vi "Configure Jitter Measurement (Clock TIE).vi"(6 "Clock TIE Slope (0: Rising)":u16(ring) items=["Rising", "Falling", "Both"], 8 "error in (no error)":errorcluster, 9 "Clock TIE Units (0: Seconds)":u16(ring) items=["Seconds", "Unit Interval"], 10 "Clock TIE Source (0: Channel 1)":u16(ring) items=["Channel 1", "Channel 2", "Channel 3", "Channel 4", "Math 1", "Math 2", "Math 3", "Math 4", "Reference Waveform 1", "Reference Waveform 2", "Reference Waveform 3", "Reference Waveform 4"], 11 "VISA resource name":refnum<visa-resource-name>) -> (0 "error out":errorcluster, 3 "VISA resource name out":refnum<visa-resource-name>)   [LabVIEW 2023, in "Keysight-DSQx3014T.lvlib"]
doc: "Enables Jitter Analysis and configures the Clock TIE (Time Interval Error) jitter measurement which compares edges in a clock signal with the edges in an ideal clock signal determined by the clock recovery feature.\n\n<b>Note:</b>\nThis VI is specific to the 6000-X Series oscilloscopes. These features are not available on other models."
uses:
  Keysight-DSQx3014T.lvlib
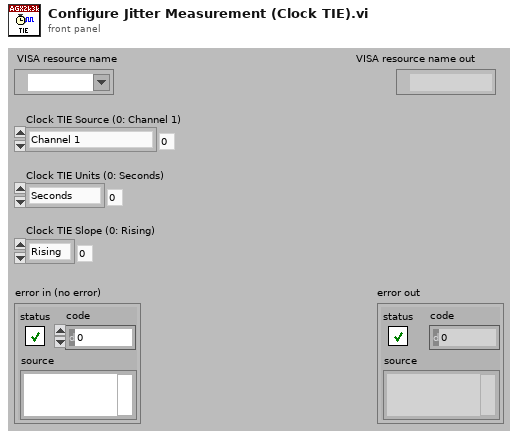
[diagram p1: front panel]
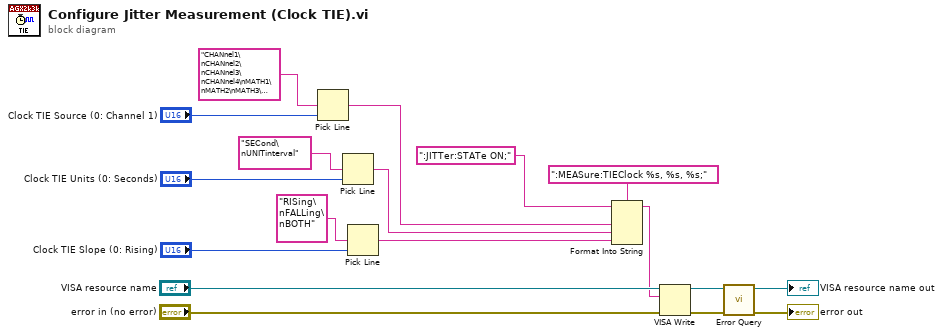
[diagram p0: block diagram]
diagram:
  n1 = Pick Line(multi-line string="CHANnel1\nCHANnel2\nCHANnel3\nCHANnel4\nMATH1\nMATH2\nMATH3\nMATH4\nWMEMory1\nWMEMory2\nWMEMory3\nWMEMory4", line index="Clock TIE Source (0: Channel 1)") -> (output string=w15:string)  [unwired: 1 in]
  n2 = Pick Line(multi-line string="SECond\nUNITinterval", line index="Clock TIE Units (0: Seconds)") -> (output string=w12:string)  [unwired: 1 in]
  n3 = Pick Line(multi-line string="RISing\nFALLing\nBOTH", line index="Clock TIE Slope (0: Rising)") -> (output string=w9:string)  [unwired: 1 in]
  n4 = Format Into String(format string=":MEASure:TIEClock %s, %s, %s;", initial string=":JITTer:STATe ON;", w15, w12, w9) -> (resulting string=w1:string)  [unwired: 1 in, 1 out]
  n5 = VISA Write(VISA resource name="VISA resource name", write buffer=w1, error in (no error)="error in (no error)") -> (VISA resource name out=w6:refnum<visa-resource-name>, error out=w4:errorcluster)  [unwired: 1 out]
  n6 = call "Error Query.vi"("error in (no error)"=w4, "VISA resource name"=w6) -> ("error out"=→"error out":errorcluster, "VISA resource name out"=→"VISA resource name out":refnum<visa-resource-name>)  [unwired: 6 in, 2 out]
